vi "Configuration Files.vi"(8 "error in (no error)":errorcluster, 11 "Node Ptr":T3 format="%.0x") -> (0 "error out":errorcluster)   [LabVIEW 2020, in "AIM ARINC 429 System Explorer.lvlib" / "Implementation.lvlib"]
uses:
  Implementation.lvlib
  <vilib>/NI VeriStand/Custom Device API/Custom Device Item Ref.ctl
  Types/Path Control.ctl
  Types/Browse Button.ctl
  Types/Configuration Files Page Data.ctl
  <vilib>/NI VeriStand/Custom Device API/Custom Device API.lvlib
  <vilib>/NI VeriStand/Custom Device Tools/Custom Device Utility Library/Custom Device Utility Library.lvlib
  Scripting/AIM/AIM ARINC 429 Scripting.lvlib
panel:
  in  "Refresh":bool
  in  "Parameters":T1
  in  "SHDocVw.IWebBrowser":refnum<k7>(container)
  in  "General Header":cluster{"Section Name":string}={"Section Name"="AIM ARINC 429 - Configuration Files"}
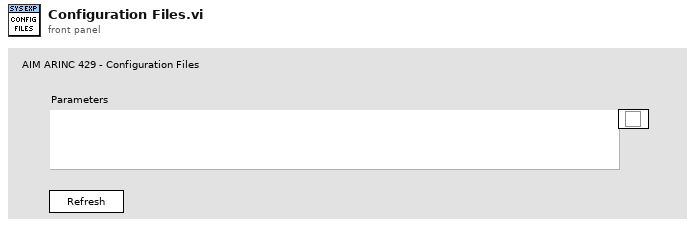
[diagram p1: front panel]
types:
  T1 = typedef "AIM ARINC 429 System Explorer.lvlib/Implementation.lvlib/Path Control.ctl" = cluster{"file path":path, "Browse":T2}
  T2 = typedef "AIM ARINC 429 System Explorer.lvlib/Implementation.lvlib/Browse Button.ctl" = bool
  T3 = typedef "Custom Device API.lvlib/Custom Device Item Ref.ctl" = u64
  T4 = typedef "AIM ARINC 429 System Explorer.lvlib/Implementation.lvlib/Configuration Files Page Data.ctl" = cluster{"Parameters":T1, "most recent parameters path":path, "custom device ref":T3, "MD5":string, "CD scripted?":bool, "parameters path ctl ref":refnum<vi>}
  T5 = typedef "Custom Device API.lvlib/Custom Device Commands.ctl" = enum16{"Default", "Item renamed", "Shutdown", "Dynamic button pressed"}
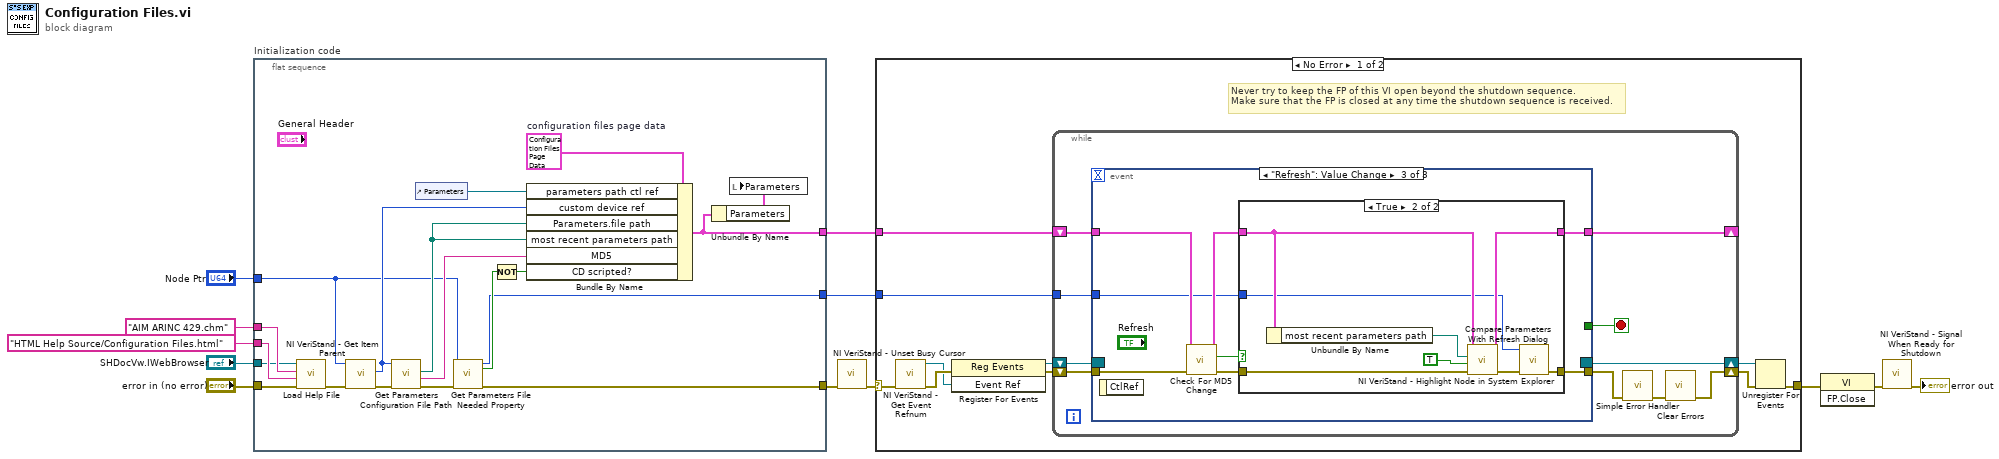
[diagram p0: block diagram]
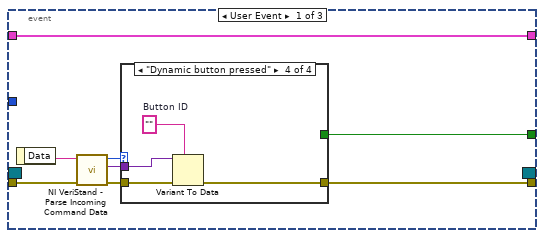
[diagram p2: hidden frame]
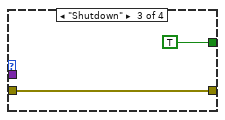
[diagram p5: hidden frame]
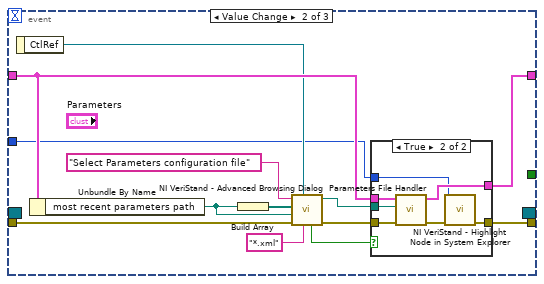
[diagram p6: hidden frame]
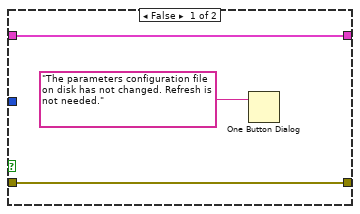
[diagram p8: hidden frame]
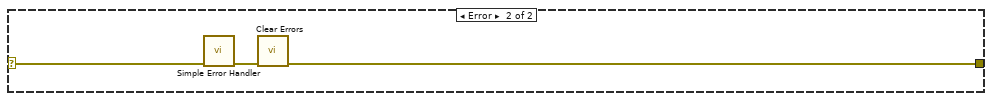
[diagram p9: hidden frame]
diagram:
  n1 = flat-sequence "Initialization code" {
    tunnel: "error in (no error)" -> [w31]
    tunnel: "Node Ptr" -> [w17]
    tunnel: [w18] -> w8
    tunnel: "SHDocVw.IWebBrowser" -> [w24]
    tunnel: "HTML Help Source/Configuration Files.html" ("CD_CHM_Section") -> [w30]
    tunnel: "AIM ARINC 429.chm" ("CD_CHM_FileName") -> [w29]
    tunnel: [w22] -> w2
    tunnel: [w13] -> w1
    frame #0 {
      w28 = T4 {"Parameters"={"file path"=path "", "Browse"=FALSE}, "most recent parameters path"=path "", "custom device ref"=0, "MD5"="", "CD scripted?"=FALSE, "parameters path ctl ref"=refnum}  # configuration files page data
      n2 = call "Load Help File.vi"("error in (no error)"=w31, "HTML File to Load"=w30, "Main CHM File"=w29, "Browser"=w24) -> ("error out"=w26:errorcluster)  [unwired: 7 in]
      n3 = call <vilib>:"NI VeriStand - Get Item Parent.vi"("error in (no error)"=w26, "Item Ref in"=w17) -> ("error out"=w14:errorcluster, "Parent Ref"=w25:T3)  [unwired: 6 in, 2 out]
      n4 = call "Get Parameters Configuration File Path.vi"("error in"=w14, "custom device ref"=w25) -> ("error out"=w19:errorcluster, "MD5 checksum"=w21:string, "parameters configuration file path"=w23:path)  [unwired: 6 in, 1 out]
      n5 = control-ref of="Parameters"() -> (w20:refnum<vi>)
      n6 = call "Get Parameters File Needed Property.vi"("error in"=w19, "configuration files ref"=w17) -> ("error out"=w18:errorcluster, "needed"=w16:bool, "configuration files ref out"=w13:T3)  [unwired: 7 in]
      n7 = Not(x=w16) -> (.not. x?=w15:bool)
      n8 = Bundle By Name(cluster=w28, "parameters path ctl ref"=w20, "custom device ref"=w25, "Parameters.file path"=w23, "most recent parameters path"=w23, "MD5"=w21, "CD scripted?"=w15) -> (w22:T4)
      n9 = Unbundle By Name(w22) -> ("Parameters"=w27:T1)
      n10 = local write "Parameters"(w27) -> ()
    }
  }
  n11 = call <vilib>:"NI VeriStand - Unset Busy Cursor.vi"("error in (no error)"=w8) -> ("error out"=w7:errorcluster)  [unwired: 10 out]
  n12 = case shown="No Error" w7 {
    selector: w7 -> [w34 w111]
    tunnel: [w38 w109] -> w12
    tunnel: w2 -> [w33 _]
    tunnel: w1 -> [w32 _]
    frame No Error {
      # "Never try to keep the FP of this VI open beyond the shutdown sequence.\nMake sure that the FP is closed at any time the shutdown sequence is received."
      n13 = call <vilib>:"NI VeriStand - Get Event Refnum.vi"("error in (no error)"=w34) -> ("error out"=w41:errorcluster, "Event Ref"=w37:refnum<user-event>)  [unwired: 9 out]
      n14 = register-events(error in=w41, w37) -> (reference out=w35:refnum<event-registration>, error out=w36:errorcluster)  [unwired: 1 in]
      n15 = while {
        shift-right: [w45] -> w39
        shift-left: w36 -> [w50]
        shift-right: [w51] -> w40
        shift-left: w35 -> [w49]
        shift-right: [w43] -> _
        shift-left: w33 -> [w44]
        tunnel: w32 -> [w42]
        stop <- w48 stop-if-true
        n16 = event shown="[2] \"Refresh\": Value Change" {
          selector: w49 -> [_ _ _]
          dyn-events: [_ _ _] -> w51
          timeout: _ -> [_ _ _]
          tunnel: w50 -> [w59 w80 w94]
          tunnel: [w55 _ _] -> w48
          tunnel: [w54 w70 w97] -> w47
          tunnel: w44 -> [w52 w74 w91]
          tunnel: [w52 w73 w96] -> w43
          tunnel: w42 -> [_ w68 w90]
          event User Event {
            n17 = event-data() -> ("Data"=w58:string)  [unwired: 1 out]
            n18 = call <vilib>:"NI VeriStand - Parse Incoming Command Data.vi"("error in (no error)"=w59, "Incoming data"=w58) -> ("error out"=w57:errorcluster, "Outgoing data"=w53:variant, "Action"=w56:T5)  [unwired: 7 out]
            n19 = case shown="\"Dynamic button pressed\"" w56 {
              tunnel: w57 -> [w60 w61 w62 w67]
              tunnel: [_ _ TRUE _] -> w55
              tunnel: [w60 w61 w62 w64] -> w54
              tunnel: w53 -> [_ _ _ w66]
              frame "Default", Default {
              }
              frame "Item renamed" {
              }
              frame "Shutdown" {
              }
              frame "Dynamic button pressed" {
                w65 = ""  # Button ID
                n20 = Variant To Data(error in=w67, type=w65, Variant=w66) -> (error out=w64:errorcluster)  [unwired: 1 out]
              }
            }
          }
          event Value Change {
            n21 = event-data() -> ("CtlRef"=w72:refnum<vi>)  [unwired: 1 out]
            n22 = Unbundle By Name(w74) -> ("most recent parameters path"=w76:path)
            n23 = Build Array(w76) -> (w78:path[])
            n24 = call <vilib>:"NI VeriStand - Advanced Browsing Dialog.vi"("File Pattern"="*.xml", "CtlRef"=w72, "error in (no error)"=w80, "Most recent path"=w76, "Paths"=w78, "Dialog Title"="Select Parameters configuration file") -> ("error out"=w75:errorcluster, "Selected file"=w71:path, "Valid?"=w69:bool)  [unwired: 2 in, 1 out]
            n25 = case shown="True" w69 {
              tunnel: w75 -> [w81 w89]
              tunnel: w74 -> [w82 w88]
              tunnel: [w82 w87] -> w73
              tunnel: w71 -> [_ w86]
              tunnel: [w81 w84] -> w70
              tunnel: w68 -> [_ w83]
              frame False {
              }
              frame True {
                n26 = call "Parameters File Handler.vi"("error in"=w89, "selected parameters file"=w86, "configuration files page data in"=w88) -> ("error out"=w85:errorcluster, "configuration files page data out"=w87:T4)  [unwired: 7 in]
                n27 = call <vilib>:"NI VeriStand - Highlight Node in System Explorer.vi"("error in (no error)"=w85, "Item Ref in"=w83) -> ("error out"=w84:errorcluster)  [unwired: 8 in, 1 out]
              }
            }
          }
          event "Refresh": Value Change {
            n28 = event-data() -> ()  [unwired: 2 out]
            n29 = call "Check For MD5 Change.vi"("error in"=w94, "configuration files page data"=w91) -> ("error out"=w93:errorcluster, "MD5 change?"=w92:bool, "configuration files page data out"=w95:T4)  [unwired: 7 in]
            n30 = case shown="True" w92 {
              tunnel: [w99 w102] -> w97
              tunnel: w93 -> [w99 w108]
              tunnel: w95 -> [w98 w107]
              tunnel: [w98 w105] -> w96
              tunnel: w90 -> [_ w101]
              frame False {
                n31 = One Button Dialog(message="The parameters configuration file on disk has not changed. Refresh is not needed.") -> ()  [unwired: 1 in, 1 out]
              }
              frame True {
                n32 = Unbundle By Name(w107) -> ("most recent parameters path"=w106:path)
                n33 = call "Compare Parameters With Refresh Dialog.vi"("error in"=w108, "refresh button"=TRUE, "selected parameters file"=w106, "configuration files page data in"=w107) -> ("error out"=w103:errorcluster, "configuration files page data out"=w105:T4)  [unwired: 6 in]
                n34 = call <vilib>:"NI VeriStand - Highlight Node in System Explorer.vi"("error in (no error)"=w103, "Item Ref in"=w101) -> ("error out"=w102:errorcluster)  [unwired: 8 in, 1 out]
              }
            }
          }
        }
        n35 = call <vilib>:"Simple Error Handler.vi"("error in (no error)"=w47) -> ("error out"=w46:errorcluster)  [unwired: 1 in, 7 out]
        n36 = call <vilib>:"Clear Errors.vi"("error in (no error)"=w46) -> ("error out"=w45:errorcluster)  [unwired: 1 in, 5 out]
      }
      n37 = Unregister For Events(event registration refnum=w40, error in=w39) -> (error out=w38:errorcluster)
    }
    frame Error {
      n38 = call <vilib>:"Simple Error Handler.vi"("error in (no error)"=w111) -> ("error out"=w110:errorcluster)  [unwired: 1 in, 7 out]
      n39 = call <vilib>:"Clear Errors.vi"("error in (no error)"=w110) -> ("error out"=w109:errorcluster)  [unwired: 1 in, 5 out]
    }
  }
  n40 = invoke class="VI" method="FP.Close"(error in=w12) -> (error out=w11:errorcluster)  [unwired: 2 in, 2 out]
  n41 = call <vilib>:"NI VeriStand - Signal When Ready for Shutdown.vi"("error in (no error)"=w11) -> ("error out"=→"error out":errorcluster)  [unwired: 10 out]
